vi "main.vi"() -> ()   [LabVIEW 2022 SP3]
uses:
  <vilib>/Utility/file.llb/Write Delimited Spreadsheet (string).vi
panel:
  out "Waveform Chart":dbl(graph)
  in  "stop":bool
  out "TIME":string
  out "DATE":string
  in  "SENSOR":dbl(slide) scale=0.0..50.0
  out "<25":bool
  out ">25":bool
  out "SENSOR IS ON":bool
  out "SENSOR VALUE":dbl
  # "REAL-TIME DATA LOGGER WITH GRAPH & ALARM"
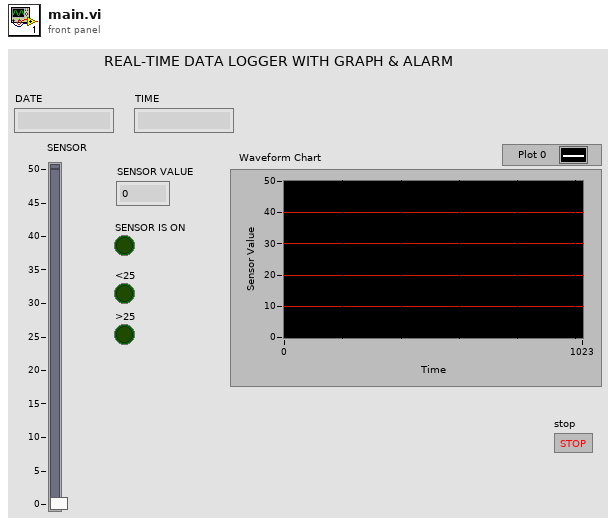
[diagram p1: front panel]
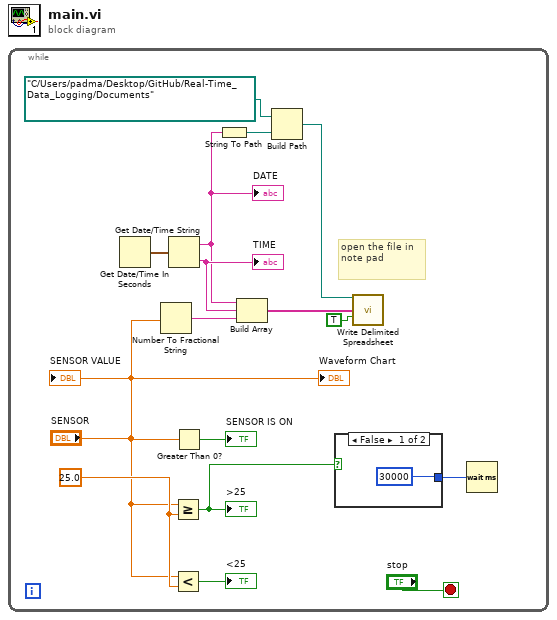
[diagram p0: block diagram]
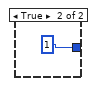
[diagram p2: hidden frame]
diagram:
  n1 = while {
    stop <- "stop" stop-if-true
    w16 = 25.0 ("y")
    # "open the file in note pad"
    n2 = Get Date/Time In Seconds() -> (seconds since 1Jan1904=w13:timestamp)
    n3 = Number To Fractional String(number="SENSOR") -> (F-format string=w11:string)  [unwired: 3 in]
    n4 = Get Date/Time String(seconds (now)=w13) -> (date string=w7:string, time string=w12:string)  [unwired: 2 in]
    "DATE" <- w7
    "TIME" <- w12
    n5 = Greater Or Equal?(x="SENSOR", y=w16) -> (x >= y?=w2:bool)
    ">25" <- w2
    n6 = Less?(x="SENSOR", y=w16) -> (x < y?=→"<25":bool)
    n7 = Greater Than 0?(x="SENSOR") -> (x > 0?=→"SENSOR IS ON":bool)
    n8 = String To Path(string=w7) -> (path=w8:path)
    n9 = Build Array(w7, w12, w11) -> (w10:string[])
    n10 = Build Path(base path=path "C:/Users/padma/Desktop/GitHub/Real-Time_Data_Logging/Documents", name or relative path=w8) -> (appended path=w9:path)
    n11 = case shown="False" w2 {
      tunnel: [u32 30000 ("milliseconds to wait") u32 1 ("milliseconds to wait")] -> w1
      frame False {
      }
      frame True {
      }
    }
    n12 = call-poly <vilib>:"Write Delimited Spreadsheet.vi"("file path (dialog if empty)"=w9, "1D data"=w10, "append to file? (new file:F)"=TRUE) -> ()  [unwired: 11 in, 2 out]
    n13 = Wait (ms)(milliseconds to wait=w1) -> ()  [unwired: 1 out]
    "SENSOR VALUE" <- "SENSOR"
    "Waveform Chart" <- "SENSOR"
  }
